vi "Is Set.vi"(8 "error in (no error)":errorcluster, 11 "Basic Type in":refnum<class "Basic Type.lvclass">) -> (0 "error out":errorcluster, 2 "Is Set":bool, 3 "Basic Type out":refnum<class "Basic Type.lvclass">)   [LabVIEW 2020, in "Protobuf RAW.lvlib" / "Basic Type.lvclass"]
uses:
  Basic Type.lvclass
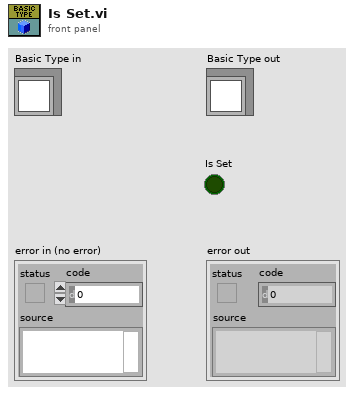
[diagram p1: front panel]
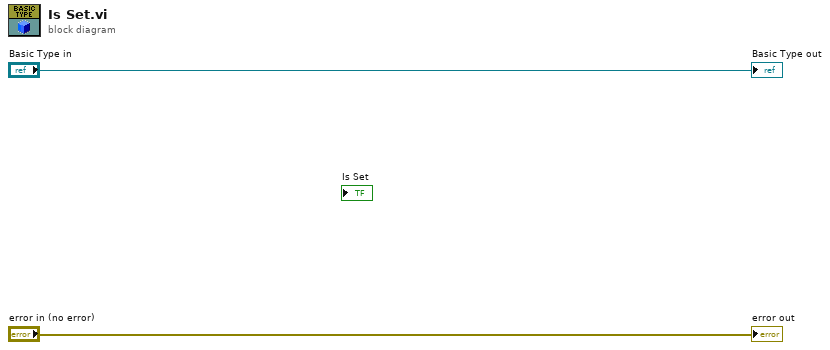
[diagram p0: block diagram]
diagram:
  "error out" <- "error in (no error)"
  "Basic Type out" <- "Basic Type in"
